vi "转矩_反馈.vi"(10 "unsigned byte array":u8[](array[numeric]), 11 "最大转矩":dbl) -> (2 "转矩反馈":dbl)   [LabVIEW 2012]
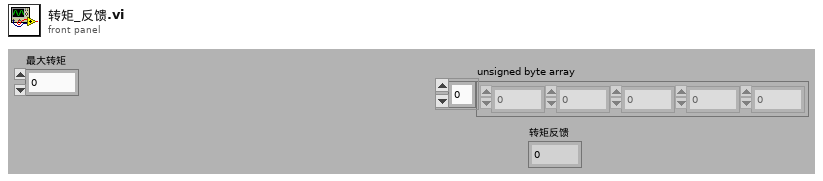
[diagram p1: front panel]
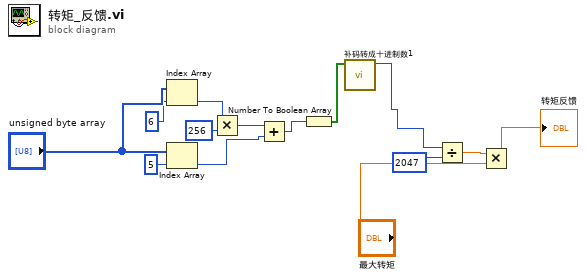
[diagram p0: block diagram]
diagram:
  n1 = Index Array(array="unsigned byte array", index=6 ("索引")) -> (element=w11:u8)
  n2 = Index Array(array="unsigned byte array", index=5 ("索引")) -> (element=w14:u8)
  n3 = Multiply(x=w11, y=u16 256) -> (x*y=w13:u16)
  n4 = Add(x=w13, y=w14) -> (x+y=w7:u16)
  n5 = Number To Boolean Array(number=w7) -> (Boolean array=w6:bool[])
  n6 = call "补码转成十进制数1.vi"("数组"=w6) -> ("x+y 2"=w5:i16)  [unwired: 10 in]
  n7 = Divide(x=w5, y=2047) -> (x/y=w3:dbl)
  n8 = Multiply(x=w3, y="最大转矩") -> (x*y=→"转矩反馈":dbl)
